vi "fetch_TCP_input.vi"(8 "error in (no error)":errorcluster) -> (0 "error out":errorcluster, 2 "data":string)   [LabVIEW 2011]
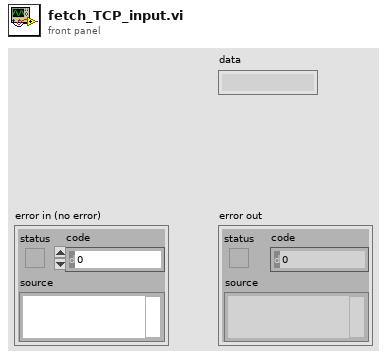
[diagram p1: front panel]
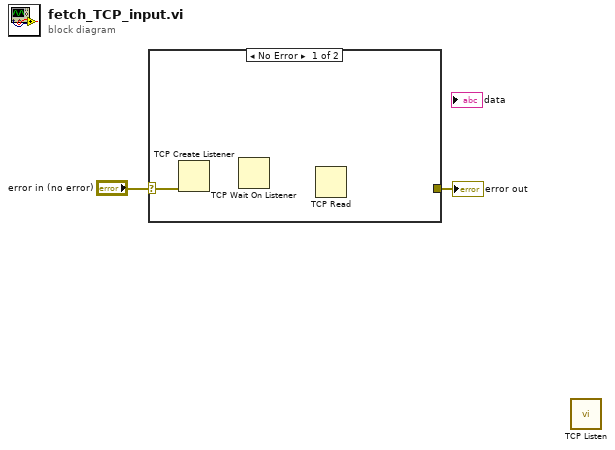
[diagram p0: block diagram]
diagram:
  n1 = case shown="No Error" "error in (no error)" {
    selector: "error in (no error)" -> [w3 w4]
    tunnel: [_ w4] -> w1
    frame No Error {
      n2 = TCP Create Listener(8:w3) -> ()  [unwired: 4 in, 3 out]
      n3 = TCP Wait On Listener() -> ()  [unwired: 4 in, 5 out]
      n4 = TCP Read() -> ()  [unwired: 5 in, 3 out]
    }
    frame Error {
    }
  }
  "error out" <- w1
  n5 = call <vilib>:"TCP Listen.vi"() -> ()  [unwired: 7 in, 5 out]
